vi "Task Init.vi"(8 "error in (no error)":errorcluster, 11 "SimTask in":refnum<class "SimTask.lvclass">) -> (0 "error out":errorcluster, 3 "SimTask out":refnum<class "SimTask.lvclass">)   [LabVIEW 2020, in "VolatusDemo.lvlib" / "SimTask.lvclass"]
uses:
  SimTask.lvclass
  SimTask.lvclass/SimTask.ctl
  Volatus/Task/Task.lvclass
  C:/dev/lv20CE/relink/lv-volatus/Volatus/Task/Task.lvclass
  C:/Program Files (x86)/National Instruments/LabVIEW 2020/vi.lib/ActorFramework/Actor/Actor.lvclass
  C:/dev/lv20CE/relink/lv-volatus/Volatus/APIRegistrationHandler/APIRegistrationHandler.lvclass
  C:/dev/lv20CE/relink/lv-volatus/Volatus/TaskStateHandler/TaskStateHandler.lvclass
  C:/dev/lv20CE/relink/lv-volatus/Volatus/VectoMessageHandler/VectoMessageHandler.lvclass
  C:/dev/lv20CE/relink/lv-volatus/VolatusDemo/SimTask/SimTask.lvclass
  lv-vecto/Vecto/Group/Group.lvclass
  C:/dev/lv20CE/relink/lv-vecto/Vecto/GroupAbstract/GroupAbstract.lvclass
  C:/dev/lv20CE/relink/lv-vecto/Vecto/Group/Group.lvclass
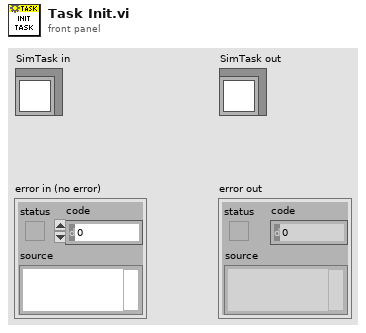
[diagram p1: front panel]
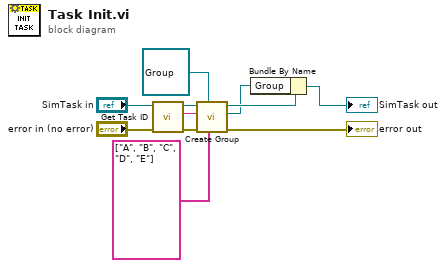
[diagram p0: block diagram]
diagram:
  n1 = call "Get Task ID.vi"("Task in"="SimTask in") -> ("Task ID"=w5:string, "Task out"=w6:refnum<class "SimTask.lvclass">)  [unwired: 9 in]
  n2 = call "Create Group.vi"("Channel Names"=string[] ["A", "B", "C", "D", "E"], "Group Type"=refnum<class "Group.lvclass"> refnum ("Vecto.lvlib:Group.lvclass"), "error in (no error)"="error in (no error)", "Group Name"=w5, "Task in"=w6) -> ("error out"=→"error out":errorcluster, "Group"=w1:refnum<class "Group.lvclass">, "Task out"=w7:refnum<class "SimTask.lvclass">)  [unwired: 4 in]
  n3 = Bundle By Name(cluster=w7, "Group"=w1) -> (→"SimTask out":refnum<class "SimTask.lvclass">)
